vi "WPI_DriverStationGetRemainingMatchTime.vi"(8 "error in (no error)":errorcluster) -> (0 "error out":errorcluster, 2 "Match Time(s)":sgl)   [LabVIEW 2017]
doc: "Returns the time remaining in the mode of the robot match. It returns -1 if the robot is disabled or in an untimed mode.\n\nThis software is licensed. Open the labview\\readme\\WPI Robotics Library Open Source License.txt file for more information."
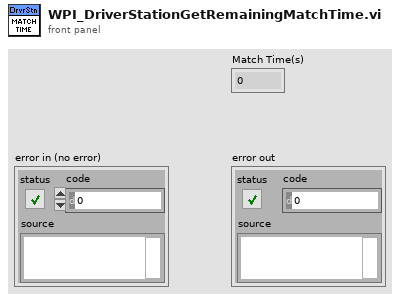
[diagram p1: front panel]
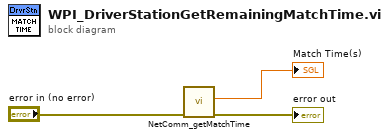
[diagram p0: block diagram]
diagram:
  n1 = call <vilib>:"NetComm_getMatchTime.vi"("error in (no error)"="error in (no error)") -> ("error out"=→"error out":errorcluster, "Match Time"=→"Match Time(s)":sgl)  [unwired: 9 in]
